vi "Initialize.vi"(7 "Channel Name":string="Setpoint.ch%d.SP", 8 "error in":errorcluster, 9 "Number of Channels":u32=1, 10 "Instance Name":string="PluginName", 11 "Power Setpoint in":refnum<class "Power Setpoint.lvclass">) -> (0 "error out":errorcluster, 3 "Power Setpoint out":refnum<class "Power Setpoint.lvclass">)   [LabVIEW 2023, in "Power Setpoint.lvclass"]
uses:
  Power Setpoint.lvclass
  Power Setpoint.lvclass/Power Setpoint.ctl
  Parents/Setpoint/Setpoint.lvclass
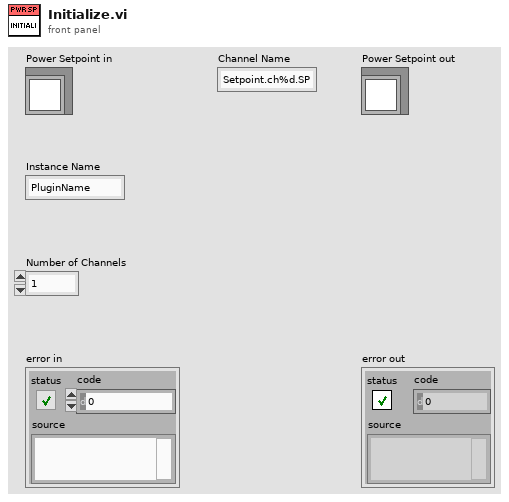
[diagram p1: front panel]
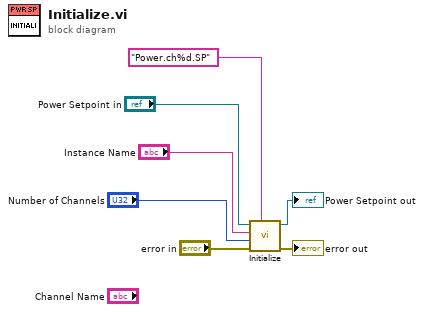
[diagram p0: block diagram]
diagram:
  n1 = call-parent "Initialize.vi"("Channel Name"="Power.ch%d.SP" ("ChannelName"), "error in"="error in", "Number of Channels"="Number of Channels", "Instance Name"="Instance Name", "Setpoint in"="Power Setpoint in") -> ("error out"=→"error out":errorcluster, "Setpoint out"=→"Power Setpoint out":refnum<class "Power Setpoint.lvclass">)  [unwired: 5 in]
